vi "Vector Product (Elements).vi"(1 "X":T1=[[1.0], [0.3]] format="%.2f", 4 "Y":T1=[[0.5], [5.0], [7.0]] format="%.2g") -> (15 "X*Y":T1=[[0.5], [1.5]] format="%.2f")   [LabVIEW 2014]
uses:
  <vilib>/Analysis/Matrix/Datatypes/RealMatrix.ctl
  <vilib>/Analysis/Matrix/NI_Matrix.lvlib
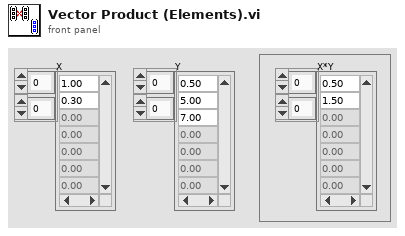
[diagram p1: front panel]
types:
  T1 = typedef "NI_Matrix.lvlib/RealMatrix.ctl" = dbl[][]
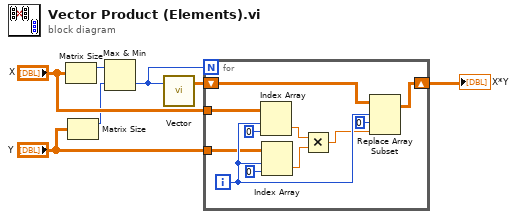
[diagram p0: block diagram]
diagram:
  n1 = Matrix Size(0:"X") -> (1:w3:i32)  [unwired: 1 out]
  n2 = Matrix Size(0:"Y") -> (1:w2:i32)  [unwired: 1 out]
  n3 = Max & Min(x=w3, y=w2) -> (min(x,y)=w1:i32)  [unwired: 1 out]
  n4 = call "Vector.vi"("length"=w1) -> ("Real Matrix (Column Vector)"=w6:T1)  [unwired: 18 in]
  n5 = for {
    N: w1 -> [_]
    tunnel: "X" -> [w15]
    shift-right: [w17] -> w5
    shift-left: w6 -> [w18]
    tunnel: "Y" -> [w8]
    i -> [w12]
    n6 = Index Array(array=w15, index (row)=w12, index (col)=0) -> (element=w11:dbl)
    n7 = Index Array(array=w8, index (row)=w12, index (col)=0) -> (element=w10:dbl)
    n8 = Multiply(x=w11, y=w10) -> (x*y=w9:dbl)
    n9 = Replace Array Subset(array=w18, new element=w9, index (row)=w12, index (col)=0 ("disabled index (col)")) -> (w17:T1)
  }
  "X*Y" <- w5
